vi "Ver 2.0.vi"() -> ()   [LabVIEW 2016]
doc: "This example VI shows how to use thermocouples to take a temperature measurement.\n\nNote:\nFor front panel measurements, make sure the Input switch is in the out position(F)\nFor plug-in card measurements, make sure the Input switch is in the in poisition(R)"
uses:
  Documents/keithley_27xx/Keithley 27XX/Public/Configure/Measurement Specific/Configure FRTD.vi
  Documents/keithley_27xx/Keithley 27XX/Public/Configure/Measurement Specific/Configure Thermocouple.vi
  Documents/keithley_27xx/Keithley 27XX/Public/Configure/Measurement Specific/Configure Thermistor.vi
  Documents/keithley_27xx/Keithley 27XX/Public/Data/Read Multiple Direct.vi
  Documents/keithley_27xx/Keithley 27XX/Keithley 27XX.lvlib
  Documents/keithley_27xx/Keithley 27XX/Public/Close.vi
panel:
  out "Case 3 T":dbl[](array[numeric])
  out "Case 2 T":dbl[](array[numeric])
  out "Case 0 T":dbl[](array[numeric])
  out "Case 3 #":dbl[](array[numeric])
  out "Case 2 #":dbl[](array[numeric])
  in  "Sample size":dbl=3.0
  in  "Sensor Type":string(combo)="Thermistor"
  in  "Delta1":dbl=1.0
  in  "Beta1":dbl=0.1
  in  "Alpha1":dbl=0.0038
  in  "Serial Configuration":T1={"Baud Rate (9600)"=9600, "Flow Control (1: XON/XOFF)"=1, "Termination Char (0:CR)"=0} {"Termination Char (0:CR)" items=["CR", "LF", "CRLF (Do not use)", "LFCR (Do not use)"]; "Flow Control (1: XON/XOFF)" items=["None", "XON/XOFF", "RTS/CTS (2701 Only)", "XON/XOFF & RTS/CTS (2701 Only)"]; "Baud Rate (9600)" items=["300"=300, "600"=600, "1200"=1200, "2400"=2400, "4800"=4800, "9600"=9600, "19.2k"=19200, "38.4k (2701 Only)"=38400, "57.6k (2701 Only)"=57600, "115.2k (2701 Only)"=115200]}
  in  "VISA resource name":refnum<visa-resource-name>="TCPIP0::192.168.69.200::1394::SOCKET"
  out "Case 0 #":dbl[](array[numeric])
  in  "Channel (101)":string="101,102,103"
  in  "Temperature (0: Celsius)":u16(ring) items=["Celsius", "Fahrenheit", "Kelvin"]
  # "*For front panel measurements, make sure the Input switch is in the out position(F)*\n  For plug-in card measurements, make sure the Input switch is in the in position(R)"
  # "© 2005 National Instruments Corporation.  ALL RIGHTS RESERVED."
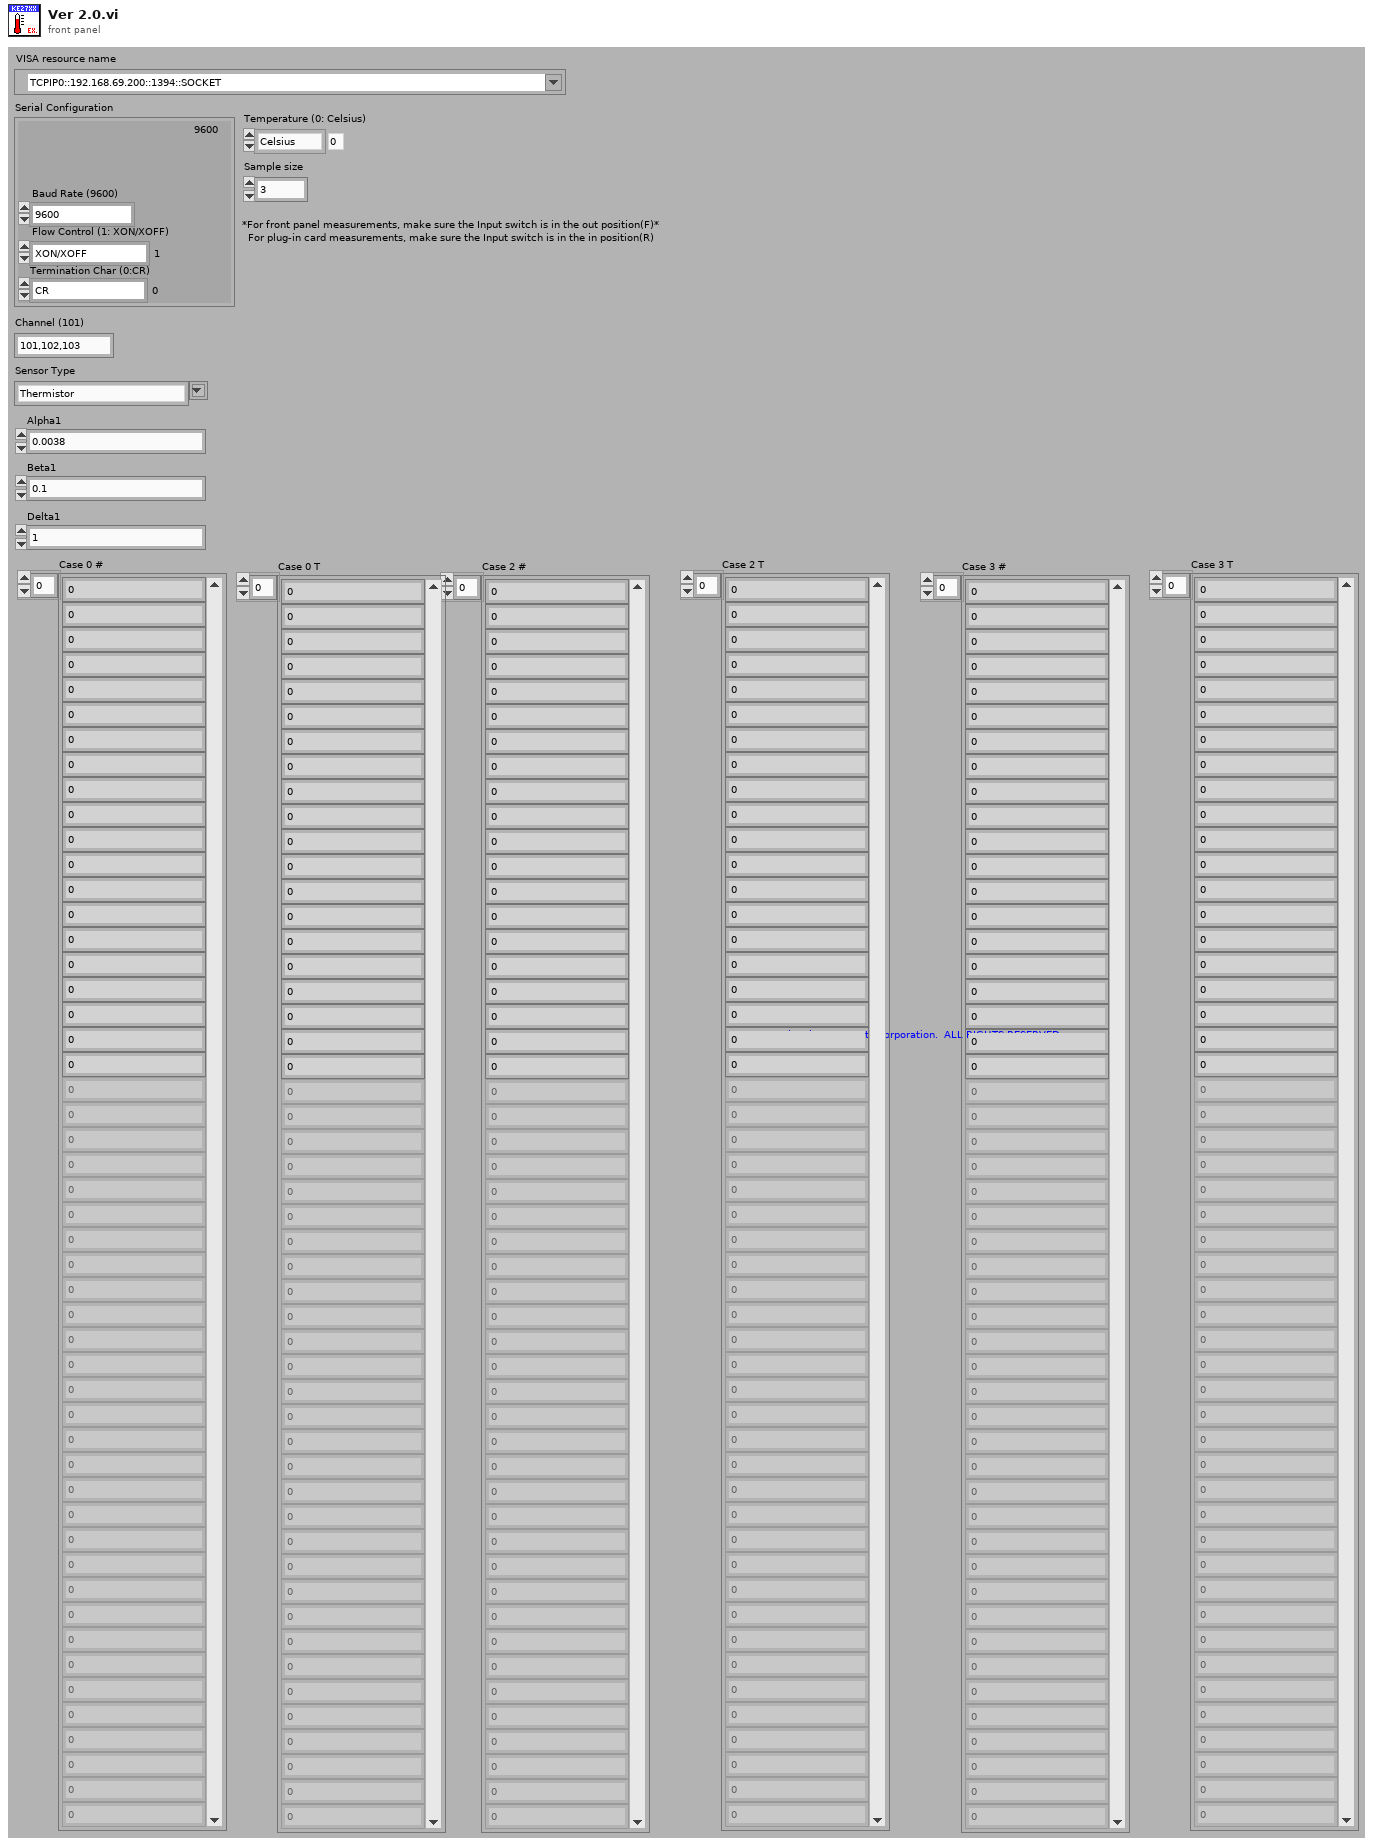
[diagram p1: front panel]
types:
  T1 = cluster{"Baud Rate (9600)":u32, "Flow Control (1: XON/XOFF)":u16, "Termination Char (0:CR)":u16}
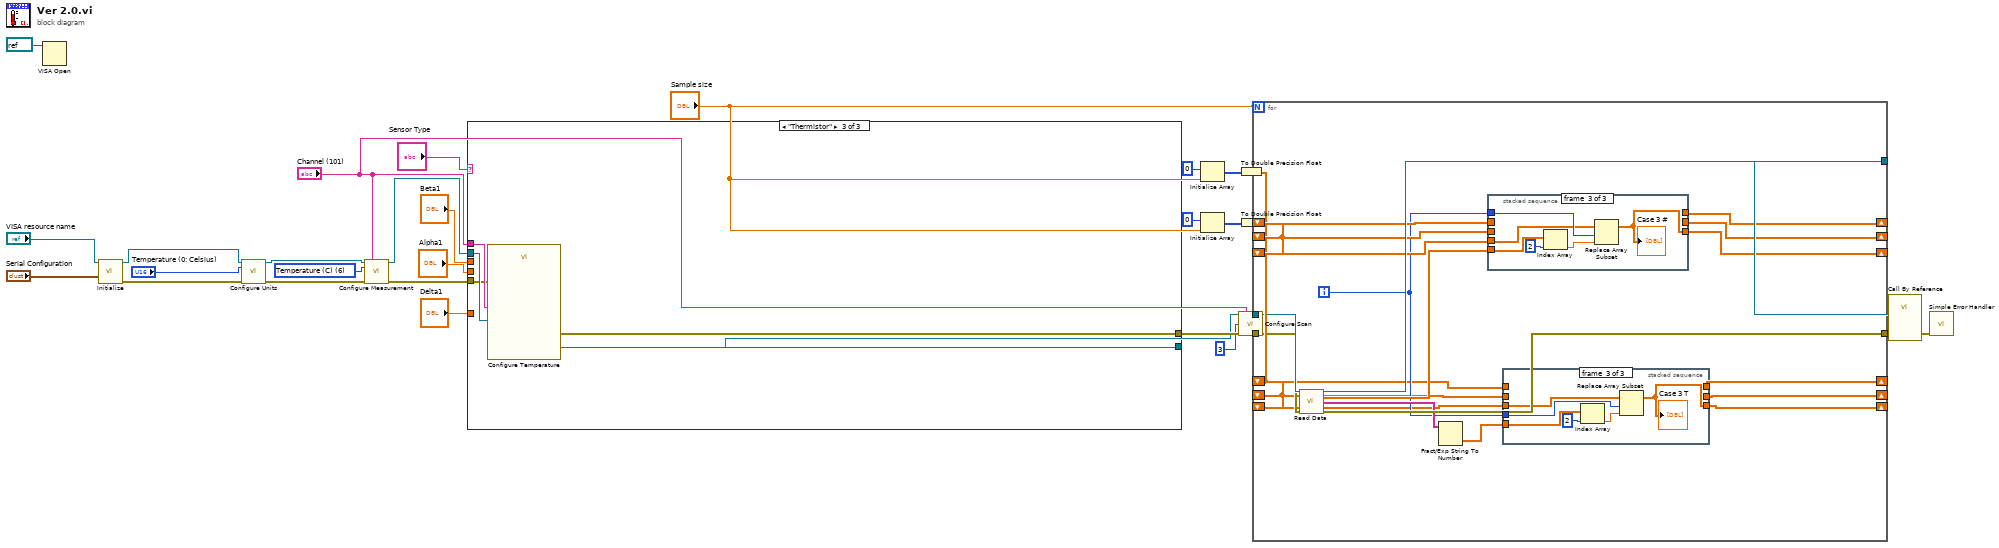
[diagram p0: block diagram]
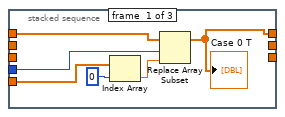
[diagram p2: hidden frame]
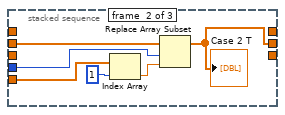
[diagram p3: hidden frame]
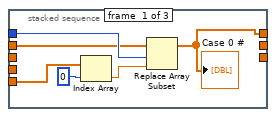
[diagram p4: hidden frame]
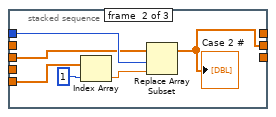
[diagram p5: hidden frame]
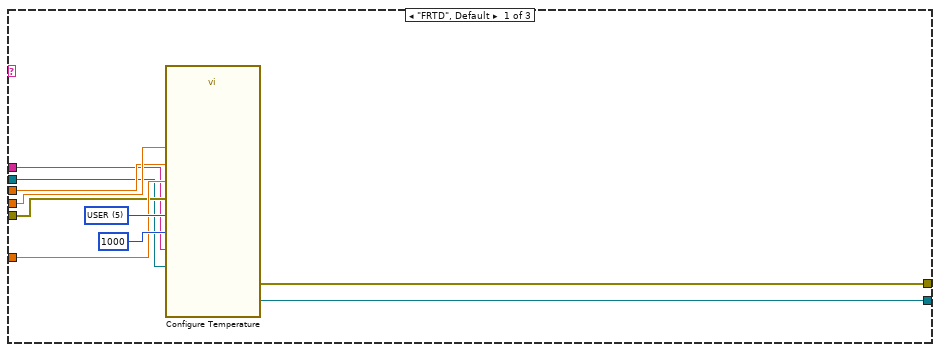
[diagram p6: hidden frame]
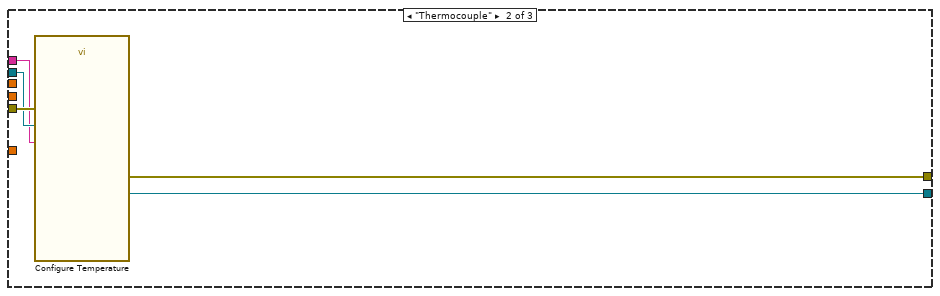
[diagram p7: hidden frame]
diagram:
  w29 = u16 6 items=["DC Voltage", "AC Voltage", "DC Current", "AC Current", "Resistance", "Four-Wire Resistance", "Temperature (C)", "Frequency", "Period", "Continuity"] ("Function (0: DC Voltage)")
  n1 = VISA Open(VISA resource name=refnum<visa-resource-name> refnum) -> ()  [unwired: 4 in, 2 out]
  n2 = call "Initialize.vi"("VISA resource name"="VISA resource name", "Serial Configuration"="Serial Configuration") -> ("VISA resource name out"=w26:refnum<visa-resource-name>, "error out"=w25:errorcluster)  [unwired: 12 in]
  n3 = call "Configure Units.vi"("VISA resource name"=w26, "Temperature (0: Celsius)"="Temperature (0: Celsius)", "error in (no error)"=w25) -> ("VISA resource name out"=w27:refnum<visa-resource-name>, "error out"=w24:errorcluster)  [unwired: 11 in]
  n4 = call "Configure Measurement.vi"("VISA resource name"=w27, "Scan List (Empty)"="Channel (101)", "Function (0: DC Voltage)"=w29, "error in (no error)"=w24) -> ("VISA resource name out"=w16:refnum<visa-resource-name>, "error out"=w17:errorcluster)  [unwired: 10 in]
  n5 = case shown="\"Thermistor\"" "Sensor Type" {
    tunnel: [w40 w45 w51] -> w22
    tunnel: [w41 w46 w50] -> w21
    tunnel: "Delta1" -> [w35 _ _]
    tunnel: "Beta1" -> [w36 _ _]
    tunnel: "Alpha1" -> [w37 _ _]
    tunnel: w17 -> [w34 w44 w47]
    tunnel: w16 -> [w33 w43 w48]
    tunnel: "Channel (101)" -> [w32 w42 w49]
    frame "FRTD", Default {
      w39 = u16 5 items=["PT100", "D100", "F100", "PT3916", "PT385", "USER"] ("FRTD Type (0: PT100)")
      n6 = call-poly "Configure Temperature.vi"("VISA resource name"=w33, "FRTD Type (0: PT100)"=w39, "error in (no error)"=w34, "Scan List (Empty)"=w32, "R Zero (100)"=1000, "Alpha (0.00385)"=w37, "Beta (0.111)"=w36, "Delta (1.507)"=w35) -> ("VISA resource name out"=w41:refnum<visa-resource-name>, "error out"=w40:errorcluster)  [unwired: 10 in]
    }
    frame "Thermocouple" {
      n7 = call-poly "Configure Temperature.vi"("VISA resource name"=w43, "error in (no error)"=w44, "Scan List (Empty)"=w42) -> ("VISA resource name out"=w46:refnum<visa-resource-name>, "error out"=w45:errorcluster)  [unwired: 15 in]
    }
    frame "Thermistor" {
      n8 = call-poly "Configure Temperature.vi"("VISA resource name"=w48, "error in (no error)"=w47, "Scan List (Empty)"=w49) -> ("VISA resource name out"=w50:refnum<visa-resource-name>, "error out"=w51:errorcluster)  [unwired: 15 in]
    }
  }
  n9 = Initialize Array(0, "Sample size") -> (w3:i32[])
  n10 = Initialize Array(0, "Sample size") -> (w11:i32[])
  n11 = call "Configure Scan.vi"("VISA resource name"=w21, "Channel List (101:110)"="Channel (101)", "Sample Count (100)"=3, "error in (no error)"=w22) -> ("VISA resource name out"=w10:refnum<visa-resource-name>, "error out"=w9:errorcluster)  [unwired: 10 in]
  n12 = To Double Precision Float(number=w3) -> (double precision float=w1:dbl[])
  n13 = To Double Precision Float(number=w11) -> (double precision float=w5:dbl[])
  n14 = for {
    N: "Sample size" -> [_]
    tunnel: w10 -> [w71]
    tunnel: w9 -> [w70]
    tunnel: [w69] -> w7
    tunnel: [w68] -> w8
    shift-right: [w65] -> _
    shift-left: w5 -> [w62]
    shift-right: [w64] -> _
    shift-left: w5 -> [w61]
    shift-right: [w66] -> _
    shift-left: w5 -> [w63]
    shift-right: [w57] -> _
    shift-left: w1 -> [w58]
    shift-right: [w55] -> _
    shift-left: w1 -> [w56]
    shift-right: [w53] -> _
    shift-left: w1 -> [w54]
    i -> [w59]
    n15 = call-poly "Read Data.vi"("VISA resource name"=w71, "error in (no error)"=w70) -> ("VISA resource name out"=w68:refnum<visa-resource-name>, "Measurement Data"=w67:dbl[], "Time Stamp"=w60:string[], "error out"=w69:errorcluster)  [unwired: 8 in, 2 out]
    n16 = Fract/Exp String To Number(string=w60) -> (number=w52:dbl[])  [unwired: 3 in, 1 out]
    n17 = stacked-sequence {
      tunnel: w59 -> [w95 w101 w107]
      tunnel: w67 -> [w94 w100 w106]
      tunnel: [w91 _ _] -> w66
      tunnel: [_ w97 _] -> w65
      tunnel: [_ _ w103] -> w64
      tunnel: w63 -> [w90 _ _]
      tunnel: w62 -> [_ w96 _]
      tunnel: w61 -> [_ _ w102]
      frame #0 {
        n18 = Index Array(array=w94, index=0) -> (element=w93:dbl)
        n19 = Replace Array Subset(array=w90, new element=w93, index=w95) -> (w91:dbl[])
        "Case 0 #" <- w91
      }
      frame #1 {
        n20 = Index Array(array=w100, index=1) -> (element=w99:dbl)
        n21 = Replace Array Subset(array=w96, new element=w99, index=w101) -> (w97:dbl[])
        "Case 2 #" <- w97
      }
      frame #2 {
        n22 = Index Array(array=w106, index=2) -> (element=w105:dbl)
        n23 = Replace Array Subset(array=w102, new element=w105, index=w107) -> (w103:dbl[])
        "Case 3 #" <- w103
      }
    }
    n24 = stacked-sequence {
      tunnel: w52 -> [w77 w83 w89]
      tunnel: [w74 _ _] -> w57
      tunnel: [_ w80 _] -> w55
      tunnel: [_ _ w86] -> w53
      tunnel: w59 -> [w73 w79 w85]
      tunnel: w58 -> [w72 _ _]
      tunnel: w56 -> [_ w78 _]
      tunnel: w54 -> [_ _ w84]
      frame #0 {
        n25 = Index Array(array=w77, index=0) -> (element=w76:dbl)
        n26 = Replace Array Subset(array=w72, new element=w76, index=w73) -> (w74:dbl[])
        "Case 0 T" <- w74
      }
      frame #1 {
        n27 = Index Array(array=w83, index=1) -> (element=w82:dbl)
        n28 = Replace Array Subset(array=w78, new element=w82, index=w79) -> (w80:dbl[])
        "Case 2 T" <- w80
      }
      frame #2 {
        n29 = Index Array(array=w89, index=2) -> (element=w88:dbl)
        n30 = Replace Array Subset(array=w84, new element=w88, index=w85) -> (w86:dbl[])
        "Case 3 T" <- w86
      }
    }
  }
  n31 = call-by-ref "?"("VISA resource name"=w8, "error in (no error)"=w7) -> ("error out"=w13:errorcluster)  [unwired: 15 in, 2 out]
  n32 = call <vilib>:"Simple Error Handler.vi"("error in (no error)"=w13) -> ()  [unwired: 4 in, 5 out]
